vi "tsdiag_can_delete_all.vi"(11 "路径输入":path) -> (3 "路径输出":path)   [LabVIEW 2019]
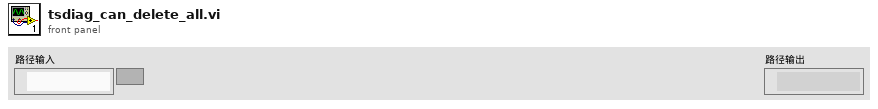
[diagram p1: front panel]
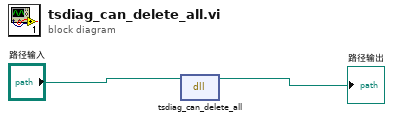
[diagram p0: block diagram]
diagram:
  n1 = dll-call lib="C:/Users/XYY/Desktop/LabView Demo/TSCAN_LB2018_V1.4_20220309/Config/TSMaster.dll" fn="tsdiag_can_delete_all"(path in="路径输入") -> (path out=→"路径输出":path)  [unwired: 3 in, 1 out]
